vi "_handle_lua_error.vi"(6 "lua status":T1=enum."LUA_ERRMEM", 8 "error in (no error)":errorcluster, 9 "error string":string) -> (0 "error out":errorcluster)   [LabVIEW 2020, in "lua.dll.lvlib"]
uses:
  lua.dll.lvlib
  lua_thread_status.ctl
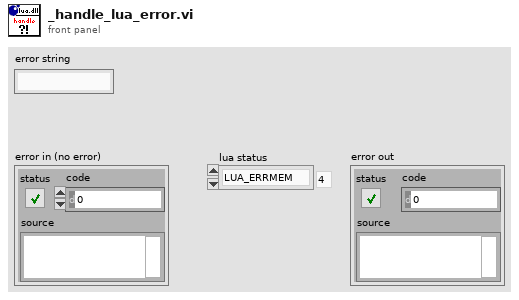
[diagram p1: front panel]
types:
  T1 = typedef "lua.dll.lvlib/lua_thread_status.ctl" = enum8{"LUA_OK", "LUA_YIELD", "LUA_ERRRUN", "LUA_ERRSYNTAX", "LUA_ERRMEM", "LUA_ERRERR"}
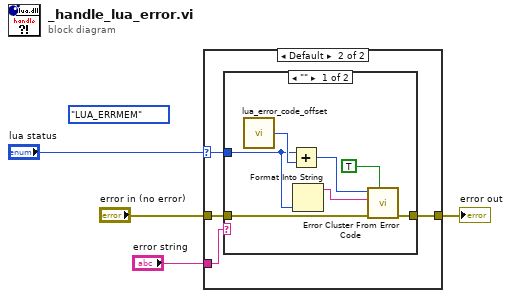
[diagram p0: block diagram]
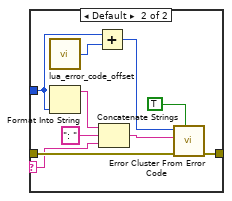
[diagram p3: hidden frame]
diagram:
  (unwired) lua_thread_status."LUA_ERRMEM" ("lua status")
  n1 = case shown="Default" "lua status" {
    selector: "lua status" -> [_ w6]
    tunnel: [w5 w9] -> w4
    tunnel: "error in (no error)" -> [w5 w8]
    tunnel: "error string" -> [_ w7]
    frame "LUA_OK", "LUA_YIELD" {
    }
    frame Default {
      n2 = case shown="\"\"" w7 {
        selector: w7 -> [_ w17]
        tunnel: w8 -> [w12 w20]
        tunnel: [w11 w19] -> w9
        tunnel: w6 -> [w10 w18]
        frame "" {
          n3 = call "lua_error_code_offset.vi"() -> ("lua error code offset"=w16:i32)
          n4 = Add(x=w10, y=w16) -> (x+y=w15:i32)
          n5 = Format Into String(w10) -> (resulting string=w13:string)  [unwired: 3 in, 1 out]
          n6 = call <vilib>:"Error Cluster From Error Code.vi"("show call chain? (False)"=TRUE, "error in (no error)"=w12, "error message (\"\")"=w13, "error code (0)"=w15) -> ("error out"=w11:errorcluster)  [unwired: 5 in]
        }
        frame Default {
          n7 = call "lua_error_code_offset.vi"() -> ("lua error code offset"=w26:i32)
          n8 = Format Into String(w18) -> (resulting string=w23:string)  [unwired: 3 in, 1 out]
          n9 = Add(x=w18, y=w26) -> (x+y=w25:i32)
          n10 = Concatenate Strings(w23, ": " ("string"), w17) -> (w21:string)
          n11 = call <vilib>:"Error Cluster From Error Code.vi"("show call chain? (False)"=TRUE, "error in (no error)"=w20, "error message (\"\")"=w21, "error code (0)"=w25) -> ("error out"=w19:errorcluster)  [unwired: 5 in]
        }
      }
    }
  }
  "error out" <- w4
